vi "ChangeFreqWFG.vi"(0 "object in":refnum<class "AD2andExtAWG.lvclass">, 2 "Freq Ch1&2":T1, 5 "error in (no error)":errorcluster) -> (14 "object out":refnum<class "AD2andExtAWG.lvclass">, 19 "error out":errorcluster)   [LabVIEW 2019, in "AD2andExtAWG.lvclass"]
uses:
  AD2andExtAWG.lvclass
  AD2andExtAWG.lvclass/AD2andExtAWG.ctl
  AFG3022B_class/AFG3022B.lvclass
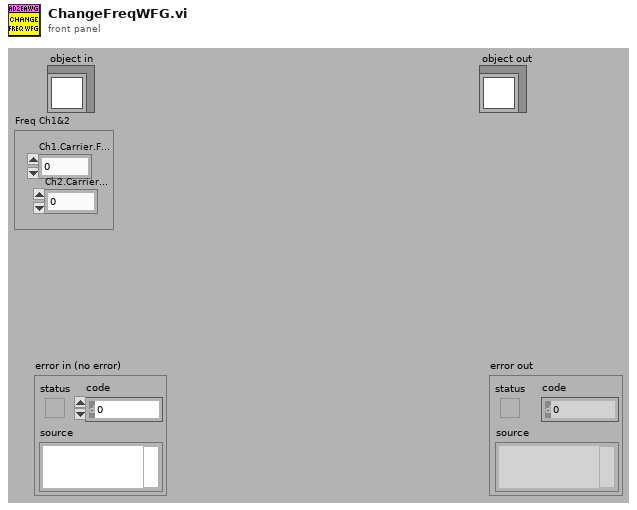
[diagram p1: front panel]
types:
  T1 = cluster{"Ch1.Carrier.Frequency (Hz)":dbl, "Ch2.Carrier.Frequency (Hz)":dbl}
  T2 = cluster{"ConfigDataCh1":cluster{"Frequency Hz (1000 Hz)":dbl, "Waveform Function (0: Sine)":u16, "Amplitude (1 Vpp)":dbl, "DC Offset (0.00 V)":dbl, "Phase Level (-1)":dbl, "Phase Unit (0: Radian)":u16}, "ConfigDataCh2":cluster{"Frequency Hz (1000 Hz)":dbl, "Waveform Function (0: Sine)":u16, "Amplitude (1 Vpp)":dbl, "DC Offset (0.00 V)":dbl, "Phase Level (-1)":dbl, "Phase Unit (0: Radian)":u16}}
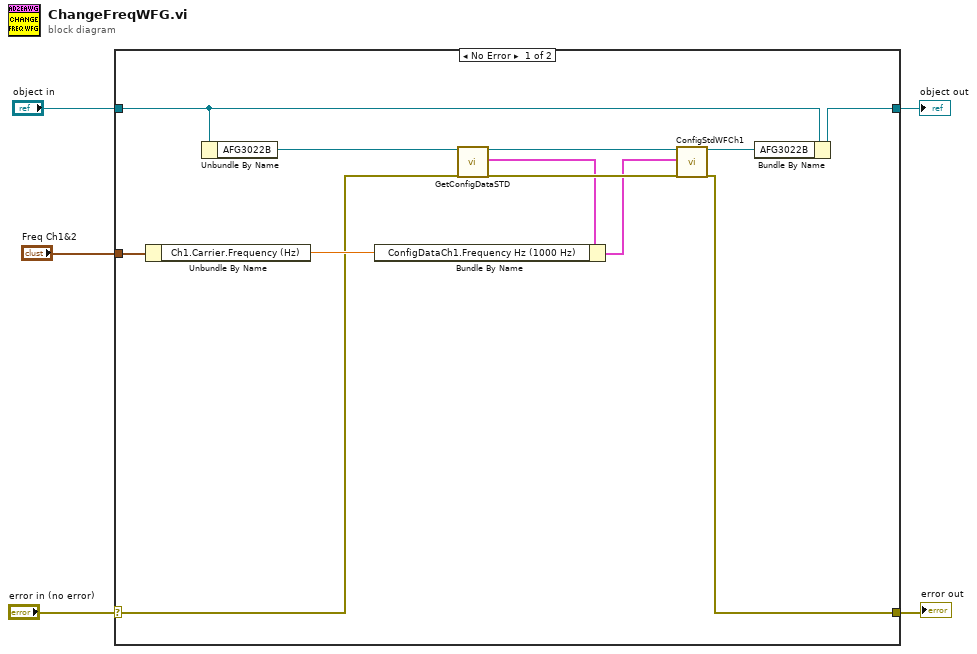
[diagram p0: block diagram]
diagram:
  n1 = case shown="No Error" "error in (no error)" {
    selector: "error in (no error)" -> [w9 w19]
    tunnel: [w8 w19] -> w4
    tunnel: [w12 w18] -> w2
    tunnel: "object in" -> [w17 w18]
    tunnel: "Freq Ch1&2" -> [w14 _]
    frame No Error {
      n2 = Unbundle By Name(w14) -> ("Ch1.Carrier.Frequency (Hz)"=w13:dbl)
      n3 = Unbundle By Name(w17) -> ("AFG3022B"=w16:refnum<class "AFG3022B.lvclass">)
      n4 = call-dynamic "GetConfigDataSTD.vi"("object in"=w16, "error in (no error)"=w9) -> ("object out"=w15:refnum<class "AFG3022B.lvclass">, "Configdatastd"=w7:T2, "error out"=w10:errorcluster)  [unwired: 15 in]
      n5 = Bundle By Name(cluster=w7, "ConfigDataCh1.Frequency Hz (1000 Hz)"=w13) -> (w6:T2)
      n6 = call-dynamic "ConfigStdWFCh1.vi"("object in"=w15, "Configdatastd"=w6, "error in (no error)"=w10) -> ("object out"=w11:refnum<class "AFG3022B.lvclass">, "error out"=w8:errorcluster)  [unwired: 15 in]
      n7 = Bundle By Name(cluster=w17, "AFG3022B"=w11) -> (w12:refnum<class "AD2andExtAWG.lvclass">)
    }
    frame Error {
    }
  }
  "error out" <- w4
  "object out" <- w2
